vi "Initialize Status Buffers.vi"(8 "error in (no error)":errorcluster, 10 "monitoring channel offsets":u64[](array[numeric]) format="%.0x", 11 "VeriStand DSF in":refnum<class "VeriStand DSF.lvclass">) -> (0 "error out":errorcluster, 3 "VeriStand DSF out":refnum<class "VeriStand DSF.lvclass">)   [LabVIEW 2017, in "DSF Engine.lvlib" / "VeriStand DSF.lvclass"]
uses:
  VeriStand DSF.lvclass
  DSF Core.lvlibp/Typedefs/DSF Data Type.ctl
  VeriStand DSF.lvclass/VeriStand DSF.ctl
  DSF Core.lvlibp/Classes/Buffer/Buffer.lvclass
  DSF Core.lvlibp/Classes/Framework/Framework.lvclass
  DSF Core.lvlibp
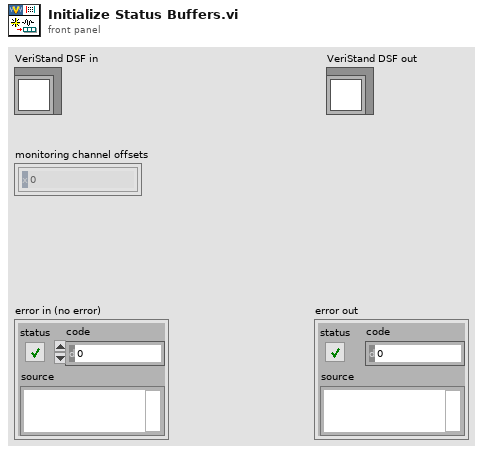
[diagram p1: front panel]
types:
  T1 = typedef "DSF Core.lvlibp/DSF Data Type.ctl" = enum8{"Bool", "SGL", "DBL", "I8", "I16", "I32", "I64", "U8", "U16", "U32", "U64"}
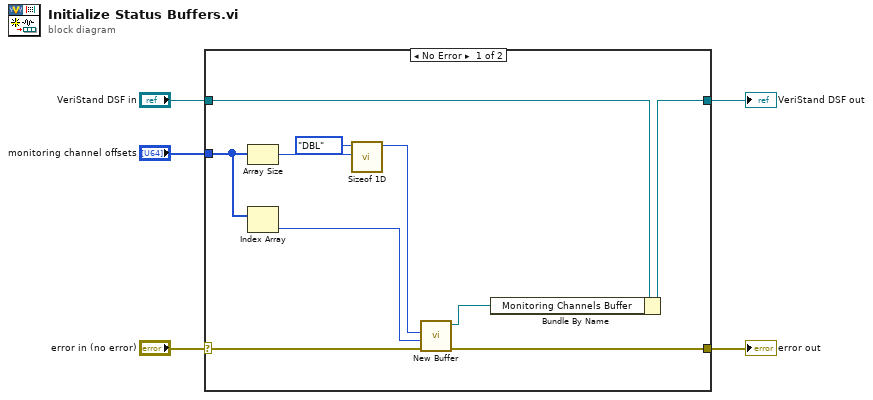
[diagram p0: block diagram]
diagram:
  n1 = case shown="No Error" "error in (no error)" {
    selector: "error in (no error)" -> [w15 w17]
    tunnel: [w9 w17] -> w4
    tunnel: "VeriStand DSF in" -> [w8 w16]
    tunnel: [w7 w16] -> w2
    tunnel: "monitoring channel offsets" -> [w12 _]
    frame No Error {
      n2 = Array Size(array=w12) -> (size(s)=w13:i32)
      n3 = Index Array(array=w12) -> (element=w11:u64)  [unwired: 1 in]
      n4 = call "Sizeof 1D.vi"("count"=w13, "data type"=DSF_Data_Type."DBL") -> ("size in bytes"=w10:u64)  [unwired: 9 in]
      n5 = call "New Buffer.vi"("error in (no error)"=w15, "buffer offset (0)"=w11, "buffer size"=w10) -> ("error out"=w9:errorcluster, "Buffer out"=w6:refnum<class "Buffer.lvclass">)  [unwired: 7 in]
      n6 = Bundle By Name(cluster=w8, "Monitoring Channels Buffer"=w6) -> (w7:refnum<class "VeriStand DSF.lvclass">)
    }
    frame Error {
    }
  }
  "error out" <- w4
  "VeriStand DSF out" <- w2
